vi "Envoyer Update.vi"(7 "Message Priority (Normal)":T1=enum."Normal" caption="Priorité des messages (normale)", 8 "error in (no error)":errorcluster caption="entrée d'erreur (pas d'erreur)", 11 "Message Enqueuer":refnum<class "Message Enqueuer.lvclass"> caption="Objet ajoutant des msgs à la file") -> (0 "error out":errorcluster caption="sortie d'erreur", 3 "Message Enqueuer out":refnum<class "Message Enqueuer.lvclass"> caption="Objet ajoutant des msgs à la file en sortie")   [LabVIEW 2015, in "Timed Loop Controller.lvlib" / "Message Update.lvclass"]
doc: "Ce VI envoie le message à un acteur."
uses:
  Message Update.lvclass
  <vilib>/ActorFramework/Message Enqueuer/Message Enqueuer.lvclass
  <vilib>/ActorFramework/Message Enqueuer/Message Priority.ctl
  <vilib>/ActorFramework/Message Enqueuer/Message Enqueuer.lvclass/Message Enqueuer.ctl
  <vilib>/ActorFramework/Message Priority Queue/Priority Enqueue.vi
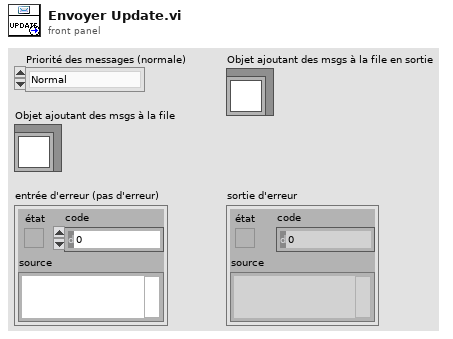
[diagram p1: front panel]
types:
  T1 = typedef "Actor Framework.lvlib/Message Enqueuer.lvclass/Message Priority.ctl" = enum16{"Low", "Normal", "High"}
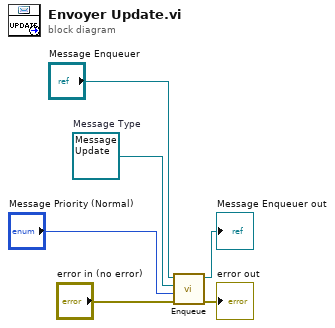
[diagram p0: block diagram]
diagram:
  w3 = refnum<class "Message Update.lvclass"> refnum  # Message Type
  n1 = call <vilib>:"Enqueue.vi"("error in (no error)"="error in (no error)", "Message Priority (Normal)"="Message Priority (Normal)", "Message"=w3, "Message Enqueuer in"="Message Enqueuer") -> ("error out"=→"error out":errorcluster, "Message Enqueuer out"=→"Message Enqueuer out":refnum<class "Message Enqueuer.lvclass">)  [unwired: 6 in]
